vi "Get Event Names.vi"(11 "Event VIs":refnum<vi>[](array[refnum])) -> (1 "Event Name":string[](array[string]), 3 "Event VIs dup":refnum<vi>[](array[refnum]))   [LabVIEW 2020, in "Panther Dashboard.lvlib"]
uses:
  Panther Dashboard.lvlib
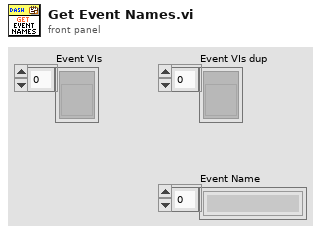
[diagram p1: front panel]
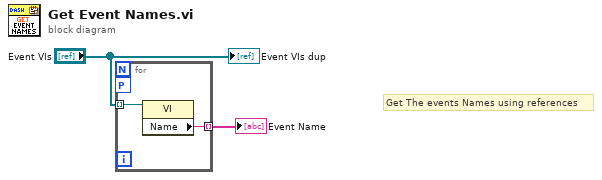
[diagram p0: block diagram]
diagram:
  # "Get The events Names using references"
  n1 = for {
    tunnel: "Event VIs" -> [w4] mode=indexing
    tunnel: [w3] -> w1 mode=indexing
    workers-P: _ -> [_]
    n2 = property class="VI"(reference=w4) -> ("Name"=w3:string)  [unwired: 1 in, 2 out]
  }
  "Event Name" <- w1
  "Event VIs dup" <- "Event VIs"
